vi "StatMon_StartWarning.vi"() -> (0 "String":string)   [LabVIEW 2019]
uses:
  Instrument_Setup.vi
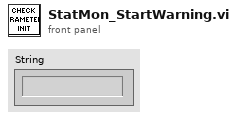
[diagram p1: front panel]
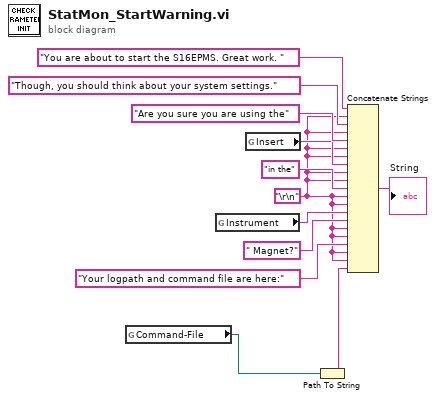
[diagram p0: block diagram]
diagram:
  w3 = "\r\n"
  n1 = global read "Instrument_Setup.vi" "Command-File"() -> (w2:path)
  n2 = global read "Instrument_Setup.vi" "Instrument"() -> (w7:string)
  n3 = global read "Instrument_Setup.vi" "Insert"() -> (w9:string)
  n4 = Path To String(path=w2) -> (string=w1:string)
  n5 = Concatenate Strings("You are about to start the S16EPMS. Great work. ", w3, "Though, you should think about your system settings.", w3, "Are you sure you are using the", w3, w3, w9, w3, w3, "in the", w3, w3, w7, " Magnet?", w3, w3, "Your logpath and command file are here:", w3, w3, w1) -> (→"String":string)
